vi "Andor_Measurement.vi"(5 "error in":errorcluster) -> (19 "error out":errorcluster)   [LabVIEW 2011]
uses:
  Program Files/National Instruments/LabVIEW 2011/resource/objmgr/daqmx.rc
  <vilib>/Utility/error.llb/DialogType.ctl
  Camera/lib/atmcd32d.llb/Error Code Enum typedef.ctl
  <vilib>/DAQmx/write.llb/DAQmx Write (Digital Bool 1Line 1Point).vi
  <vilib>/DAQmx/create/channels.llb/DAQmx Create Channel (DO-Digital Output).vi
  <vilib>/DAQmx/read.llb/DAQmx Read (Digital Bool 1Line 1Point).vi
  Kinetics/vi/GlobalSettings.vi
  Utilities/controls/ctlSeqFNs_PI_SysNr.ctl
  <vilib>/DAQmx/configure/trigger.llb/DAQmx Start Trigger (Digital Edge).vi
  <vilib>/DAQmx/create/channels.llb/DAQmx Create Channel (CO-Pulse Generation-Frequency).vi
  <vilib>/DAQmx/configure/timing.llb/DAQmx Timing (Implicit).vi
  <vilib>/DAQmx/create/channels.llb/DAQmx Create Channel (DI-Digital Input).vi
panel:
  in  "out":T1
  in  "valsZaxisMeasurement":T2
  out "error out 2":errorcluster
  out "last":i32
  out "first":u32
  out "pic2 2":dbl[][](graph)
  out "pic2":dbl[][](graph)
  out "intens":i32[][](graph)
  in  "PictureInfo 2":T3
  in  "Intensity DataInit":i32[][](graph)
  in  "Intensitätsdiode":dbl[](array[numeric])
  in  "Binning":T4
  in  "PictureInfo":T3
  out "y num vorgae":i32
  out "z vorgabe":i32
  out "z num":i32
  out "y num":i32
  out "x num":i32
  out "Intensity Graph Out Andor Null 2":i32[][](graph)
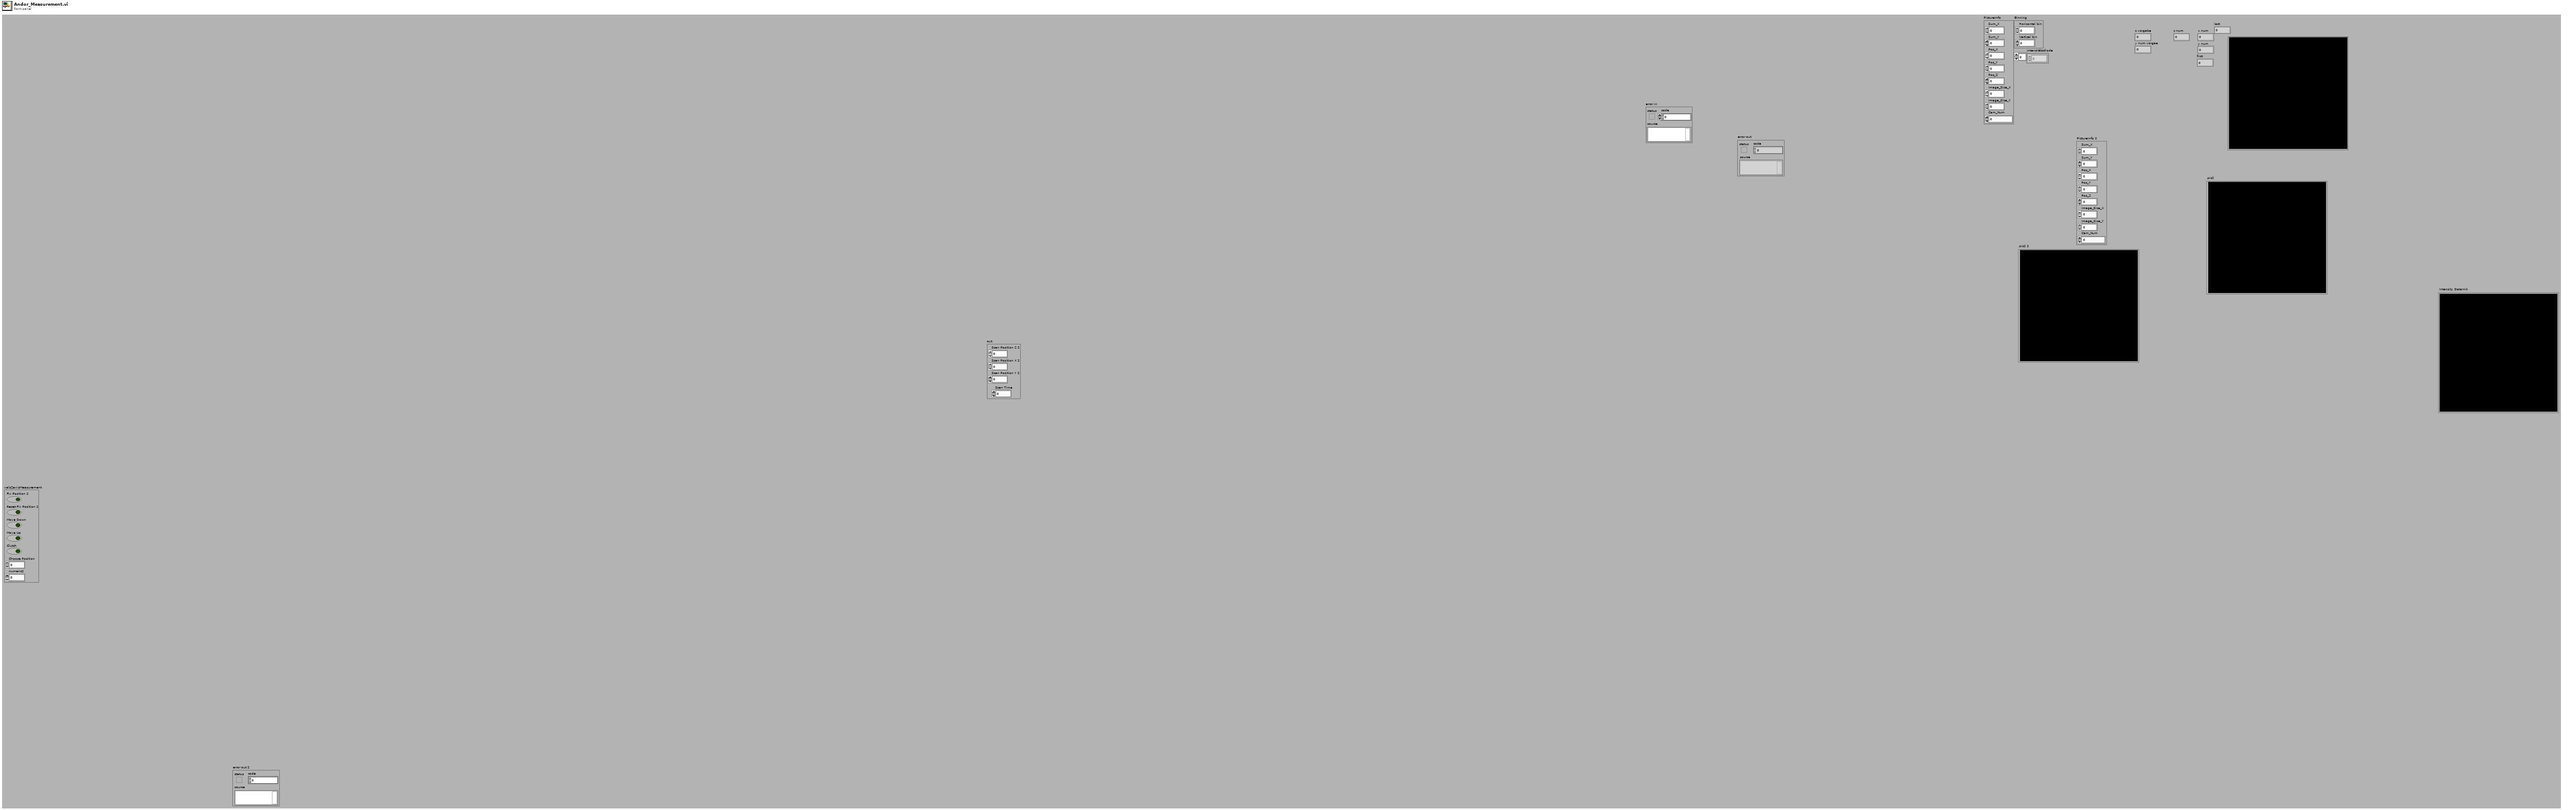
[diagram p1: front panel]
types:
  T1 = cluster{"Scan Position Z 2":dbl, "Scan Position X 2":dbl, "Scan Position Y 2":dbl, "Scan Time":dbl}
  T2 = cluster{"Fix Position 2":bool, "Reset Fix Position 2":bool, "Move Down":bool, "Move Up":bool, "Clutch":bool, "Choose Position":dbl, "numeric2":dbl}
  T3 = cluster{"Sum_X":i32, "Sum_Y":i32, "Pos_X":dbl, "Pos_Y":dbl, "Pos_Z":dbl, "Image_Size_X":dbl, "Image_Size_Y":dbl, "Cam_Num":i32}
  T4 = cluster{"Horizontal bin":i32, "Vertical bin":i32}
  T5 = typedef "ctlSeqFNs_PI_SysNr.ctl" = enum16{"Zero", "E517", "E710"}
  T6 = typedef "E517_Termination_character.ctl" = enum16{"LF", "CR", "LFCR", "CRLF"}
  T7 = typedef "E517_Controller_names.ctl" = enum16{"None", "Analog", "C-702", "C-843", "C-843.PM", "C-844", "C-848", "C-865", "C-866", "C-867", "C-880", "E-516", "E-517", "E-710", "E-712", "E-725", "E-753", "E-755", "E-761", "E-816", "E-861", "F-206", "M-840", "M-850", "M-8X0", "Mercury"}
  T8 = typedef "E517_Available_DLLs.ctl" = u16
  T9 = typedef "E517_Available_DLL_interfaces.ctl" = u16
  T10 = typedef "E517_Available_interfaces.ctl" = u16
  T11 = cluster{"Main-Global-Config out":cluster{"Global-Config":cluster{"DLL device ID's":i32[], "DLL Interface\nConfiguration":cluster{"DLL for Device":T8, "DLL Interface":T9, "Parameter":string}[], "Interface configuration":cluster{"RS232 Portnumber":i32, "Timeout":i32, "RS232 Baud rate":u32, "Interface":T10, "GPIB Bus":i32, "GPIB Address":i32, "GPIB Mode":i32}[], "Flow control":cluster{"input XON/XOFF":bool, "input HW Handshake":bool, "input alt HW HShk":bool, "output XON/XOFF":bool, "output HW Handshake":bool, "output alt HW HShk":bool, "XOFF byte ":u8, "XON byte":u8, "parity error byte":u16}[], "Bit settings and parity":cluster{"data bits":u16, "stop bits":enum16{"1 bit", "1.5 bits", "2 bits"}, "parity":enum16{"no parity", "odd parity", "even parity", "mark parity", "space parity"}}[], "TCP/IP Configuration":cluster{"Host address/name":string, "Port":i32, "Board":i32}[], "VISA Resource name":refnum<visa-resource-name>[], "Termination character":T6[], "Syntax":enum16{"GCS 1.0", "GCS 2.0"}[], "Logging mode":bool[], "Log file ref. no":refnum<file>[], "System no.":i32}, "DaisyChain configuration":cluster{"No. of devices":i32, "Port ID":i32, "Devices":string[], "Description":string}[], "System":cluster{"Conn. axes":string[], "Controller name":T7}[]}, "Axis-Status":cluster{"Online status (Array)?":bool[], "WG running?":bool[], "Servo status?":bool[]}, "Identification":string, "Conn. Axes":string[], "Position":dbl[], "+/- movement range":dbl[]}
  T12 = typedef "Error Code Enum typedef.ctl" = enum32{"N/A (0)", "DRV_ERROR_CODES", "DRV_SUCCESS", "DRV_VXDNOTINSTALLED", "DRV_ERROR_SCAN", "DRV_ERROR_CHECK_SUM", "DRV_ERROR_FILELOAD", "DRV_UNKNOWN_FUNC", "DRV_ERROR_VXD_INIT", "DRV_ERROR_ADDRESS", "DRV_ERROR_PAGELOCK", "DRV_ERROR_PAGEUNLOCK", "DRV_ERROR_BOARDTEST", "DRV_ERROR_ACK", "DRV_ERROR_UP_FIFO", "DRV_ERROR_PATTERN", "N/A (16)", "DRV_ACQUISITION_ERRORS", "DRV_ACQ_BUFFER", "DRV_ACQ_DOWNFIFO_FULL", "DRV_PROC_UNKONWN_INSTRUCTION", "DRV_ILLEGAL_OP_CODE", "DRV_KINETIC_TIME_NOT_MET", "DRV_ACCUM_TIME_NOT_MET", "DRV_NO_NEW_DATA", "N/A (25)", "DRV_SPOOLERROR", "N/A (27)", "N/A (28)", "N/A (29)", "N/A (30)", "N/A (31)", "N/A (32)", "DRV_TEMPERATURE_CODES", "DRV_TEMPERATURE_OFF", "DRV_TEMPERATURE_NOT_STABILIZED", "DRV_TEMPERATURE_STABILIZED", "DRV_TEMPERATURE_NOT_REACHED", "DRV_TEMPERATURE_OUT_RANGE", "DRV_TEMPERATURE_NOT_SUPPORTED", "DRV_TEMPERATURE_DRIFT", "N/A (41)", "N/A (42)", "N/A (43)", "N/A (44)", "N/A (45)", "N/A (46)", "N/A (47)", "N/A (48)", "DRV_GENERAL_ERRORS", "DRV_INVALID_AUX", "DRV_COF_NOTLOADED", "DRV_FPGAPROG", "DRV_FLEXERROR", "DRV_GPIBERROR", "N/A (55)", "N/A (56)", "N/A (57)", "N/A (58)", "N/A (59)", "N/A (60)", "N/A (61)", "N/A (62)", "N/A (63)", "DRV_DATATYPE", "DRV_DRIVER_ERRORS", "DRV_P1INVALID", "DRV_P2INVALID", "DRV_P3INVALID", "DRV_P4INVALID", "DRV_INIERROR", "DRV_COFERROR", "DRV_ACQUIRING", "DRV_IDLE", "DRV_TEMPCYCLE", "DRV_NOT_INITIALIZED", "DRV_P5INVALID", "DRV_P6INVALID", "DRV_INVALID_MODE", "DRV_INVALID_FILTER", "DRV_I2CERRORS", "DRV_I2CDEVNOTFOUND", "DRV_I2CTIMEOUT", "DRV_P7INVALID", "N/A (84)", "N/A (85)", "N/A (86)", "N/A (87)", "N/A (88)", "N/A (89)", "DRV_IOCERROR", "DRV_VRMVERSIONERROR"}
  T13 = cluster{"exposure":sgl, "accumulate":sgl, "kinetic":sgl}[]
  T14 = cluster{"exposure":sgl, "accumulate":sgl, "kinetic":sgl}
  T15 = cluster{"Initial delay":dbl, "Duty Cycle":dbl, "Frequency":dbl, "sample mode":i32, "Number Of Pulses":i32, "SrcToCtrOutTriggerForCamera":tag, "CtrOutTriggerForCamera":tag}
  T16 = cluster{"X-Min":dbl, "X-Len":dbl, "Y-Min":dbl, "Y-Len":dbl, "X-Delta":dbl, "Y-Delta ":dbl}
  T17 = cluster{"3d Layers_Num":dbl, "3d Start_Pos  Start":dbl, "3d Step_Delta_Layer":dbl}
  T18 = cluster{"Picture_Parameter_Out":enum16{"Maximized", "Averaged", "Normalized"}, "SavingMode":enum32{"Confocal", "HighRes", "Video", "Picture", "IntensityTrace", "Test"}}
  T19 = enum32{"Confocal", "HighRes", "Video", "Picture", "IntensityTrace", "Test"}
  T20 = typedef "DialogType.ctl" = u16
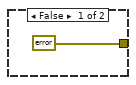
[diagram p3: hidden frame]
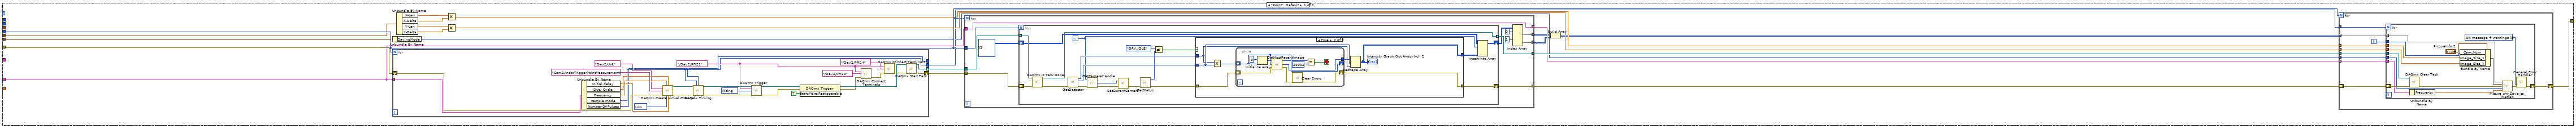
[diagram p4: hidden frame]
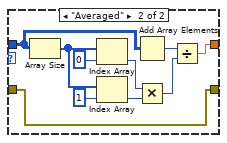
[diagram p9: hidden frame]
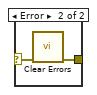
[diagram p10: hidden frame]
diagram:
  (unwired) ctlSeqFNs_PI_SysNr."E710" ("DeviceNr.")
  n1 = case shown="\"Point\", Default" {
    selector: _ -> [_ _]
    tunnel: _ -> [w45 _]
    tunnel: [w39 w46] -> w12
    tunnel: _ -> [w44 _]
    tunnel: [w42 _] -> w4
    frame "Point", Default {
      n2 = Unbundle By Name(w44) -> ("Conn. Axes"=w43)
      n3 = call "MVR.vi"("System no."=w42, "Axes to move"=w43, "Position values"=dbl[] [100.0, 100.0], "No.of digits"=i16 4, "error in"=w45) -> ("error out"=w39:errorcluster)  [unwired: 14 in]
    }
    frame "XDArea" {
    }
  }
  "error out 2" <- w12
  n4 = call "MeasurementAktivFCG.vi"("error in"="error in", "Set_Get"=enum16{"Set", "Get"}."Set", "Value"=TRUE) -> ("error out"=w9:errorcluster)  [unwired: 7 in, 1 out]
  n5 = call "HeidenhainValsPre.vi"(1:"valsZaxisMeasurement", 2:TRUE ("Reset Fix Position"), 5:w9) -> (6:w3)  [unwired: 5 in]
  n6 = call "SetupAquisitionParameters.vi"("error in"=w3) -> ("error out"=w13:errorcluster)  [unwired: 18 in]
  n7 = call "SetGetMeasurement_TypeFGV.vi"("error in"=w13, "FGV_Control"=enum16{"Set", "Get"}."Get") -> ("error out"=w20:errorcluster, "Measurement Type 2"=w22:enum16{"Point", "XDArea"})  [unwired: 8 in]
  n8 = call "ConfigureCamera.vi"("error in"=w20, "Set_Get"=enum16{"Set", "Get"}."Get") -> ("error out"=w19:errorcluster, "out"=w17:cluster{"Hbin":i32, "Vbin":i32, "ExpTime":sgl})  [unwired: 8 in]
  n9 = Unbundle By Name(w17) -> ("Vbin"=w16:i32, "Hbin"=w15:i32)
  n10 = call "GetAvailableCameras.vi"("error in (no error)"=w19) -> ("error out"=w25:errorcluster, "totalCameras"=w14:i32, "DLL error code"=w37:u32)  [unwired: 2 in]
  n11 = call "SetAndorOnlineOfflineFGV.vi"("error in"=w25, "Set_Get"=enum16{"Set", "Get"}."Get") -> ("error out"=w6:errorcluster, "andor 1"=w29:bool, "andor 0"=w30:bool)  [unwired: 7 in]
  n12 = Not(x=w30) -> (.not. x?=w27:bool)
  n13 = global read "GlobalSettings.vi" "scanner global out"() -> (w5:T11)
  n14 = Boolean To (0,1)(Boolean=w27) -> (0, 1=w31:i16)
  n15 = Not(x=w29) -> (.not. x?=w28:bool)
  n16 = Subtract(x=w14, y=w31) -> (x-y=w32:i32)
  n17 = Boolean To (0,1)(Boolean=w28) -> (0, 1=w33:i16)
  n18 = Subtract(x=w32, y=w33) -> (x-y=w23:i32)
  n19 = Not Equal To 0?(x=w23) -> (x != 0?=w34:bool)
  n20 = Equal?(x=w37, y=u32 20002) -> (x = y?=w35:bool)
  n21 = Or(x=w34, y=w35) -> (x .or. y?=w24:bool)
  n22 = case shown="True" w24 {
    tunnel: w23 -> [_ w79]
    tunnel: w22 -> [_ w72]
    tunnel: [errorcluster {"status"=FALSE, "code"=0, "source"="noCameraAtSetupAcquisitionParameters"} ("error out") w78] -> w21
    tunnel: w16 -> [_ w65]
    tunnel: w15 -> [_ w64]
    tunnel: w6 -> [_ w51]
    tunnel: w5 -> [_ w48]
    tunnel: ctlSeqFNs_PI_SysNr."E710" ("DeviceNr.") -> [_ w49]
    frame False {
    }
    frame True {
      n23 = call "GetConfiguratioOfCamera.vi"("error in"=w51, "Set_Get"=enum16{"Set", "Get"}."Get") -> ("error out"=w62:errorcluster, "out"=w55:T13)  [unwired: 8 in]
      n24 = Index Array(array=w55, index #1=0 ("index"), index #2=1 ("index")) -> (element #1=w58:T14, element #2=w59:T14)
      n25 = Unbundle By Name(w58) -> ("exposure"=w60:sgl)
      n26 = Unbundle By Name(w59) -> ("exposure"=w61:sgl)
      n27 = Max & Min(x=w60, y=w61) -> (max(x,y)=w50:sgl)  [unwired: 1 out]
      n28 = call "3D_Distance_FGV.vi"("error in"=w62, "FGV_Control"=enum16{"Set", "Get"}."Get") -> ("error out"=w52:errorcluster)  [unwired: 8 in, 1 out]
      n29 = call "TriggerPointMeasurement.vi"("error in"=w52, "Set_Get"=enum16{"Set", "Get"}."Get") -> ("error out"=w75:errorcluster, "out"=w76:T15)  [unwired: 8 in]
      n30 = call "RoiSelectionCoordinates.vi"("error in"=w75, "FGV_Control"=enum16{"Set", "Get"}."Get") -> ("error out"=w71:errorcluster, "ROI Coordinates out"=w73:T16)  [unwired: 8 in]
      n31 = call "3D_Distance_FGV.vi"("error in"=w71, "FGV_Control"=enum16{"Set", "Get"}."Get") -> ("error out"=w68:errorcluster, "3D out"=w69:T17)  [unwired: 8 in]
      n32 = call "Save_Picture_Parameter_FGV.vi"("error in"=w68, "FGV_Control"=enum16{"Set", "Get"}."Get") -> ("error out"=w63:errorcluster, "Picture_Parameter_Out"=w66:T18)  [unwired: 8 in]
      n33 = case shown="\"XDArea\"" w72 {
        tunnel: w79 -> [w95 w324]
        tunnel: [w101 w261] -> w78
        tunnel: w63 -> [w99 w209]
        tunnel: w76 -> [w94 _]
        tunnel: w73 -> [w90 w210]
        tunnel: w69 -> [_ w207]
        tunnel: w66 -> [w92 w302]
        tunnel: w65 -> [_ w292]
        tunnel: w64 -> [_ w293]
        tunnel: w50 -> [_ w208]
        tunnel: w49 -> [_ w206]
        tunnel: w48 -> [_ w205]
        frame "Point", Default {
          n34 = Unbundle By Name(w92) -> ("SavingMode"=w91:T19)
          n35 = for {
            N: w95 -> [_]
            shift-right: [w188] -> w100
            shift-left: w99 -> [w176]
            tunnel: w94 -> [w186]
            tunnel: [w187] -> w98 mode=indexing
            tunnel: [w178] -> w80
            tunnel: [w177] -> _
            w180 = tag "/Dev2/PFI21" ("source")
            w197 = 10280 items=["Rising"=10280, "Falling"=10171] ("Trigger Edge")
            w200 = 10214 items=["High"=10192, "Low"=10214] ("Idle State")
            n36 = Unbundle By Name(w186) -> ("Initial delay"=w189:dbl, "Duty Cycle"=w191:dbl, "Frequency"=w190:dbl, "sample mode"=w177:i32, "Number Of Pulses"=w178:i32)
            n37 = call-poly <vilib>:"DAQmx Create Virtual Channel.vi"("frequency"=w190, "duty cycle"=w191, "counter"=tag "Dev2/ctr6", "name to assign"="Cam1AndorTriggerPointMeasurement", "error in"=w176, "idle state"=w200, "initial delay"=w189) -> ("task out"=w201:refnum<k21>, "error out"=w202:errorcluster)  [unwired: 7 in]
            n38 = call-poly <vilib>:"DAQmx Timing.vi"("task/channels in"=w201, "sample mode"=w177, "samples per channel"=w178, "error in"=w202) -> ("task out"=w199:refnum<k21>, "error out"=w198:errorcluster)  [unwired: 10 in]
            n39 = call-poly <vilib>:"DAQmx Trigger.vi"("task/channels in"=w199, "source"=w180, "edge"=w197, "error in"=w198) -> ("task out"=w195:refnum<k21>, "error out"=w194:errorcluster)  [unwired: 10 in]
            n40 = property class="DAQmx Trigger"(reference=w195, error in=w194, "Start:More:Retriggerable"=TRUE) -> (reference out=w192:refnum<k21>, error out=w183:errorcluster)
            n41 = call <vilib>:"DAQmx Connect Terminals.vi"("source terminal"=w180, "destination terminal"=tag "/Dev2/PFI20", "error in"=w183) -> ("error out"=w182:errorcluster)  [unwired: 12 in]
            n42 = call <vilib>:"DAQmx Connect Terminals.vi"("source terminal"=w180, "destination terminal"=tag "/Dev2/PFI24", "error in"=w182) -> ("error out"=w181:errorcluster)  [unwired: 12 in]
            n43 = call <vilib>:"DAQmx Start Task.vi"("task/channels in"=w192, "error in"=w181) -> ("task out"=w187:refnum<k21>, "error out"=w188:errorcluster)  [unwired: 12 in]
          }
          n44 = Unbundle By Name(w90) -> ("X-Len"=w89:dbl, "X-Delta"=w88:dbl, "Y-Len"=w86:dbl, "Y-Delta"=w87:dbl)
          n45 = Multiply(x=w89, y=w88) -> (x*y=w85:dbl)
          n46 = Multiply(x=w86, y=w87) -> (x*y=w84:dbl)
          n47 = for {
            N: w80 -> [_]
            tunnel: w100 -> [w113]
            tunnel: w98 -> [w112]
            tunnel: [w111] -> w97
            tunnel: [w110] -> w96
            tunnel: w95 -> [w109]
            tunnel: w94 -> [w108]
            tunnel: [w108] -> w93
            tunnel: [w104] -> w83 mode=indexing
            tunnel: [w102] -> w82 mode=indexing
            n48 = for {
              N: w109 -> [_]
              shift-right: [w122] -> w111
              shift-left: w113 -> [w118]
              tunnel: [w119] -> w110 mode=indexing
              tunnel: w112 -> [w120] mode=indexing
              shift-right: [w116] -> w106
              shift-left: i32[][][] [] ("array") -> [w115]
              i -> [w117]
              n49 = call <vilib>:"DAQmx Is Task Done.vi"("task/channels in"=w120, "error in"=w118) -> ("task out"=w119:refnum<k21>, "error out"=w123:errorcluster)  [unwired: 11 in, 1 out]
              n50 = call "GetDetector.vi"("error in (no error)"=w123) -> ("error out"=w126:errorcluster, "ypixels"=w124:i32, "xpixels"=w125:i32)  [unwired: 3 in, 1 out]
              n51 = call "GetCameraHandle.vi"("error in (no error)"=w126, "cameraIndex"=w117) -> ("error out"=w131:errorcluster, "cameraHandle"=w132:i32)  [unwired: 1 in, 1 out]
              n52 = call "SetCurrentCamera.vi"("error in (no error)"=w131, "cameraHandle"=w132) -> ("error out"=w130:errorcluster)  [unwired: 1 out]
              n53 = call "GetStatus.vi"("error in (no error)"=w130) -> ("error out"=w129:errorcluster, "status"=w127:T12)  [unwired: 2 in, 1 out]
              n54 = Not Equal?(x=Error_Code_Enum_typedef."DRV_IDLE" ("status"), y=w127) -> (x != y?=w121:bool)
              n55 = case shown="True" w121 {
                tunnel: [w133 w134] -> w122
                tunnel: w129 -> [w133 w138]
                tunnel: w125 -> [_ w136]
                tunnel: w124 -> [_ w137]
                tunnel: [_ w135] -> w114
                frame False {
                }
                frame True {
                  n56 = Multiply(x=w136, y=w137) -> (x*y=w139:i32)
                  n57 = while {
                    tunnel: [w144] -> w140
                    shift-right: [w147] -> w134
                    shift-left: w138 -> [w141]
                    shift-right: [w145] -> _
                    shift-left: w139 -> [w145]
                    stop <- w149 stop-if-true
                    n58 = Initialize Array(0 ("element"), w145) -> (w146:i32[])
                    n59 = call "GetMostRecentImage.vi"("error in (no error)"=w141, "size"=w145, "array"=w146) -> ("error out"=w142:errorcluster, "array"=w144:i32[], "DLL error code"=w143:u32)
                    n60 = call <vilib>:"Clear Errors.vi"("error in (no error)"=w142) -> ("error out"=w147:errorcluster)  [unwired: 6 in]
                    n61 = Equal?(x=w143, y=u32 20002) -> (x = y?=w149:bool)
                  }
                  n62 = Reshape Array(w140, w137, w136) -> (w135:i32[][])
                  "Intensity Graph Out Andor Null 2" <- w135
                }
              }
              n63 = Insert Into Array(array=w115, index (dim 0)=w117, new element=w114) -> (w116:i32[][][])  [unwired: 2 in]
            }
            n64 = Index Array(array=w106, index (dim 0) #1=0 ("index"), index (dim 0) #2=1 ("index (page)")) -> (element #1=w104:i32[][], element #2=w102:i32[][])  [unwired: 4 in]
          }
          n65 = Build Array(w83, w82) -> (w81:i32[][][][])
          n66 = for {
            N: w95 -> [_]
            shift-right: [w151] -> w101
            shift-left: w97 -> [w160]
            tunnel: w96 -> [w159] mode=indexing
            tunnel: w93 -> [w158]
            tunnel: w91 -> [w157]
            tunnel: w85 -> [w155]
            tunnel: w84 -> [w154]
            tunnel: w81 -> [w153] mode=indexing
            tunnel: w80 -> [w152]
            i -> [w156]
            n67 = for {
              N: w152 -> [_]
              tunnel: w159 -> [w173]
              tunnel: w158 -> [w172]
              tunnel: w157 -> [w168]
              tunnel: w156 -> [w165]
              tunnel: w155 -> [w164]
              tunnel: w154 -> [w163]
              tunnel: w153 -> [w162] mode=indexing
              shift-right: [w161] -> w151
              shift-left: w160 -> [w174]
              w175 = T20 3 items=["no dialog", "OK message", "continue or stop message", "OK message + warnings", "continue/stop + warnings"] ("type of dialog (OK msg:1)")
              n68 = call <vilib>:"DAQmx Clear Task.vi"("task in"=w173, "error in"=w174) -> ("error out"=w171:errorcluster)  [unwired: 13 in]
              n69 = Unbundle By Name(w172) -> ("Frequency"=w169:dbl)
              n70 = Bundle By Name(cluster="PictureInfo 2", "Cam_Num"=w165, "Image_Size_X"=w164, "Image_Size_Y"=w163) -> (w166:T3)
              n71 = call "Picture_shr_Save_to_matlab.vi"("DataIn"=w162, "PictureInfo"=w166, "error in"=w171, "SavingMode"=w168, "Freuquency"=w169) -> ("error out"=w170:errorcluster)  [unwired: 10 in]
              n72 = call <vilib>:"General Error Handler.vi"("type of dialog (OK msg:1)"=w175, "error in (no error)"=w170) -> ("error out"=w161:errorcluster)  [unwired: 9 in, 4 out]
            }
          }
        }
        frame "XDArea" {
          w217 = 0 ("X0")
          w252 = TRUE ("All axes?")
          w307 = T20 0 items=["no dialog", "OK message", "continue or stop message", "OK message + warnings", "continue/stop + warnings"] ("type of dialog (OK msg:1)")
          w312 = T20 0 items=["no dialog", "OK message", "continue or stop message", "OK message + warnings", "continue/stop + warnings"] ("type of dialog (OK msg:1)")
          n73 = Unbundle By Name(w210) -> ("X-Min"=w222:dbl, "Y-Min"=w245:dbl, "X-Len"=w218:dbl, "Y-Len"=w250:dbl, "Y-Delta"=w248:dbl, "X-Delta"=w223:dbl)
          n74 = Divide(x=w250, y=w248) -> (x/y=w249:dbl)
          n75 = Divide(x=w218, y=w223) -> (x/y=w221:dbl)
          n76 = call "Calc_frequency.vi"("ExitationTime In"=w208, "X-length"=w218, "CamTolerance"=1.1, "frequency in"=5000, "error in"=w209, "X-Delta"=w223) -> ("Wavepoints"=w212:dbl, "N"=w211:dbl, "TriggerLineCamWavepoints"=w216:dbl[], "divisor out"=w215:i32, "Array"=w214:u8[], "error out"=w220:errorcluster)  [unwired: 4 in]
          n77 = Unbundle By Name(w205) -> ("Conn. Axes"=w213:string[])
          n78 = call "Calc_WaveformGenerator.vi"("Scan parameters"=w215, "Wavepoint"=w213, "Trigger value 2"=w212, 3:w214, "wave table rate/ms"=w217, "System no."=w206, "scan time for 1 line/ms"=w217, 7:w216, 8:w211, 9:w217, 10:w211, "error in 2"=w220, 12:w218) -> ("error out 2"=w219:errorcluster)  [unwired: 2 in]
          n79 = call "ONT?.vi"("System no."=w206, "Axes to query"=w213, "All axes?"=w252, "Axis identifier?"=w252, "error in"=w219) -> ("error out"=w257:errorcluster)  [unwired: 13 in, 1 out]
          n80 = call "TMN?.vi"("System no."=w206, "Axes to query"=w213, "All axes?"=w252, "Axis identifier?"=w252, "error in"=w257) -> ("error out"=w258:errorcluster)  [unwired: 13 in, 1 out]
          n81 = call "TMX?.vi"("System no."=w206, "Axes to query"=w213, "All axes?"=w252, "Axis identifier?"=w252, "error in"=w258) -> ("error out"=w253:errorcluster)  [unwired: 13 in, 1 out]
          n82 = for {
            N: w249 -> [_]
            shift-right: [w398] -> _
            shift-left: w245 -> [w399]
            tunnel: [w398] -> w256 mode=indexing
            shift-right: [w397] -> w254
            shift-left: w253 -> [w397]
            tunnel: w248 -> [w396]
            n83 = Add(x=w399, y=w396) -> (x+y=w398:dbl)
          }
          n84 = Unbundle By Name(w207) -> ("3d Layers_Num"=w251:dbl, "3d Start_Pos  Start"=w244:dbl, "3d Step_Delta_Layer"=w247:dbl)
          n85 = Divide(x=w251, y=w247) -> (x/y=w246:dbl)
          n86 = for {
            N: w246 -> [_]
            shift-right: [w394] -> _
            shift-left: w244 -> [w395]
            tunnel: [w394] -> w255 mode=indexing
            shift-right: [w393] -> w243
            shift-left: w254 -> [w393]
            tunnel: w247 -> [w392]
            n87 = Add(x=w395, y=w392) -> (x+y=w394:dbl)
          }
          n88 = Unbundle By Name(w302) -> ("Picture_Parameter_Out"=w269:enum16{"Maximized", "Averaged", "Normalized"}, "SavingMode"=w296:T19)
          n89 = Unbundle By Name(w207) -> ("3d Step_Delta_Layer"=w277:dbl, "3d Layers_Num"=w279:dbl, "3d Start_Pos  Start"=w270:dbl)
          n90 = call "StartTimingDIO_ScannerStage.vi"(2:w243) -> (5:w240, 7:w239, 11:w241, 13:w234, 14:w237, 15:w235, 16:w204, 17:w236, 18:w242, 19:w238)  [unwired: 9 in]
          n91 = Divide(x=w279, y=w277) -> (x/y=w278:dbl)
          n92 = for {
            N: w246 -> [_]
            tunnel: w213 -> [w350]
            tunnel: w206 -> [w349]
            tunnel: w256 -> [w348]
            tunnel: w222 -> [w347]
            tunnel: w255 -> [w346] mode=indexing
            shift-right: [w345] -> w233
            shift-left: _ -> [_]
            tunnel: w249 -> [w344]
            tunnel: w242 -> [w343]
            tunnel: w241 -> [w342]
            tunnel: w240 -> [w341]
            tunnel: w239 -> [w340]
            tunnel: w238 -> [w339]
            tunnel: w237 -> [w338]
            tunnel: w236 -> [w337]
            tunnel: w235 -> [w336]
            tunnel: w234 -> [w335]
            tunnel: [w334] -> w232
            tunnel: [w333] -> w231
            tunnel: [w332] -> w230
            tunnel: [w331] -> w229
            tunnel: [w330] -> w228
            tunnel: [w329] -> w227
            tunnel: [w328] -> w226
            tunnel: [w327] -> w225
            tunnel: [w326] -> w224
            tunnel: w221 -> [w325]
            n93 = for {
              N: w344 -> [_]
              shift-right: [_] -> w345
              shift-left: _ -> [_]
              tunnel: w349 -> [w352]
              tunnel: w350 -> [w353]
              tunnel: w348 -> [w389] mode=indexing
              tunnel: w347 -> [w388]
              tunnel: w346 -> [w387]
              tunnel: w343 -> [w372]
              tunnel: w342 -> [w371]
              tunnel: w341 -> [w370]
              tunnel: w340 -> [w369]
              tunnel: w339 -> [w368]
              tunnel: w338 -> [w367]
              tunnel: w337 -> [w366]
              tunnel: w336 -> [w365]
              tunnel: w335 -> [w364]
              tunnel: [w363] -> w334
              tunnel: [w362] -> w333
              tunnel: [w361] -> w332
              tunnel: [w360] -> w331
              tunnel: [w359] -> w330
              tunnel: [w358] -> w329
              tunnel: [w357] -> w328
              tunnel: [w356] -> w327
              tunnel: [w355] -> w326
              tunnel: w325 -> [w354]
              w385 = TRUE ("Axis identifier?")
              n94 = Build Array(w388, w389, w387) -> (w390:dbl[])
              n95 = call "MOV.vi"("System no."=w352, "Axes to move"=w353, "Position values"=w390, "No.of digits"=i16 1) -> ("error out"=w351:errorcluster)  [unwired: 15 in]
              n96 = call "TriggerTheCamera.vi"(0:w372, 1:w368, 2:w367, 3:w366, 4:w365, 5:w364, 6:w354, "error out 2"=w351, 8:w371, 10:w370, 12:w369) -> (14:w355, 16:w356, 18:w357, 21:w358, 22:w359, 23:w360, 24:w361, 25:w362, 26:w363, "error out"=w386:errorcluster)  [unwired: 7 in]
              n97 = call "POS?.vi"("System no."=w352, "Axes to query"=w353, "All axes?"=w385, "Axis identifier?"=w385, "error in"=w386) -> ("Position"=w380:dbl[], "error out"=w384:errorcluster)  [unwired: 13 in]
              n98 = Index Array(array=w380, index #1=0 ("index"), index #2=1 ("index"), index #3=2 ("index")) -> (element #1=w378:dbl, element #2=w376:dbl, element #3=w374:dbl)
              n99 = Bundle By Name(cluster="out", "Scan Position X 2"=w378, "Scan Position Y 2"=w376, "Scan Position Z 2"=w374) -> (w381:T1)
              n100 = call "ScanPosition_FGV.vi"("error in"=w384, "FGV_Control"=enum16{"Set", "Get"}."Set", "in"=w381) -> ("error out"=w383:errorcluster)  [unwired: 7 in, 1 out]
              n101 = call <vilib>:"Clear Errors.vi"("error in (no error)"=w383) -> ()  [unwired: 6 in, 1 out]
            }
          }
          n102 = call-poly <vilib>:"DAQmx Create Virtual Channel.vi"("lines"=tag "Dev2/port0/line10", "name to assign"="CamStartInputTimer", "error in"=w204) -> ("task out"=w287:refnum<k21>, "error out"=w265:errorcluster)  [unwired: 11 in]
          n103 = call-poly <vilib>:"DAQmx Create Virtual Channel.vi"("lines"=tag "Dev2/port0/line5", "name to assign"="CameraStartInput", "error in"=w265) -> ("task out"=w316:refnum<k21>, "error out"=w321:errorcluster)  [unwired: 11 in]
          n104 = call-poly <vilib>:"DAQmx Create Virtual Channel.vi"("lines"=tag "Dev2/port0/line6", "name to assign"="CameraReadOutDoneX", "error in"=w321) -> ("task out"=w314:refnum<k21>, "error out"=w306:errorcluster)  [unwired: 11 in]
          n105 = call <vilib>:"DAQmx Start Task.vi"("task/channels in"=w316, "error in"=w306) -> ("task out"=w315:refnum<k21>, "error out"=w266:errorcluster)  [unwired: 12 in]
          n106 = call <vilib>:"DAQmx Start Task.vi"("task/channels in"=w287, "error in"=w266) -> ("task out"=w286:refnum<k21>, "error out"=w267:errorcluster)  [unwired: 12 in]
          n107 = call-poly <vilib>:"DAQmx Write.vi"("task/channels in"=w286, "data"=FALSE, "error in"=w267) -> ("task out"=w285:refnum<k21>, "error out"=w280:errorcluster)  [unwired: 10 in, 1 out]
          n108 = Unbundle By Name(w210) -> ("X-Min"=w275:dbl, "Y-Min"=w298:dbl, "X-Len"=w273:dbl, "Y-Len"=w271:dbl, "X-Delta"=w276:dbl, "Y-Delta"=w281:dbl)
          n109 = call "CameraReady.vi"("error in"=w280, "Set_Get"=enum16{"Set", "Get"}."Set", "Value"=TRUE) -> ("error out"=w203:errorcluster)  [unwired: 7 in, 1 out]
          n110 = Divide(x=w273, y=w276) -> (x/y=w274:dbl)
          n111 = Divide(x=w271, y=w281) -> (x/y=w272:dbl)
          n112 = for {
            N: w278 -> [w441]
            tunnel: w324 -> [w443]
            tunnel: w272 -> [w434]
            tunnel: w274 -> [w442]
            shift-right: [w431] -> w310
            shift-left: w203 -> [w436]
            tunnel: w315 -> [w440]
            tunnel: w314 -> [w439]
            tunnel: [w438] -> w308
            tunnel: [w437] -> w309
            tunnel: [w435] -> w300
            tunnel: [w434] -> w299
            tunnel: [w433] -> w305
            tunnel: w269 -> [w432]
            tunnel: w285 -> [w425]
            tunnel: [w426] -> w284
            tunnel: [w421] -> w264 mode=indexing
            tunnel: [w420] -> w263 mode=indexing
            i -> [w433]
            n113 = for {
              N: w434 -> [w498]
              tunnel: w443 -> [w506]
              shift-right: [w504] -> w429
              shift-left: w436 -> [w483]
              tunnel: w440 -> [w505]
              tunnel: w439 -> [w496]
              tunnel: [w493] -> w438
              tunnel: [w503] -> w437
              tunnel: w442 -> [w502]
              tunnel: [w492] -> w435
              tunnel: w432 -> [w491]
              tunnel: [w490] -> w430
              tunnel: w425 -> [w481]
              tunnel: [w489] -> w426
              tunnel: [w488] -> w424
              tunnel: [w487] -> w423
              tunnel: [w469] -> w421 mode=indexing
              tunnel: [w468] -> w420 mode=indexing
              i -> [w473]
              n114 = call-poly <vilib>:"DAQmx Write.vi"("task/channels in"=w481, "data"=FALSE, "error in"=w483) -> ("task out"=w482:refnum<k21>, "error out"=w478:errorcluster)  [unwired: 10 in, 1 out]
              n115 = call-poly <vilib>:"DAQmx Write.vi"("task/channels in"=w496, "data"=FALSE, "timeout"=10.0, "error in"=w478) -> ("task out"=w495:refnum<k21>, "error out"=w497:errorcluster)  [unwired: 9 in, 1 out]
              n116 = while {
                tunnel: w497 -> [w511]
                tunnel: w505 -> [w515]
                tunnel: [w514] -> w499
                tunnel: w482 -> [w513]
                tunnel: [w512] -> w485
                tunnel: [w509] -> w477
                stop <- w507 stop-if-true
                n117 = call-poly <vilib>:"DAQmx Read.vi"("task/channels in"=w515, "error in"=w511) -> ("task out"=w514:refnum<k21>, "data"=w507:bool, "error out"=w510:errorcluster)  [unwired: 11 in]
                n118 = call-poly <vilib>:"DAQmx Write.vi"("task/channels in"=w513, "data"=TRUE, "error in"=w510) -> ("task out"=w512:refnum<k21>, "error out"=w509:errorcluster)  [unwired: 10 in, 1 out]
              }
              n119 = call-poly <vilib>:"DAQmx Write.vi"("task/channels in"=w485, "data"=FALSE, "error in"=w477) -> ("task out"=w486:refnum<k21>, "error out"=w484:errorcluster)  [unwired: 10 in, 1 out]
              n120 = for {
                N: w506 -> [_]
                shift-right: [w519] -> w500
                shift-left: w484 -> [w537]
                tunnel: w495 -> [w535]
                tunnel: [w536] -> w493
                tunnel: w499 -> [w536]
                tunnel: [w535] -> w494
                tunnel: w502 -> [w516]
                tunnel: [w516] -> w492
                tunnel: w491 -> [w534]
                tunnel: [w529] -> w490 mode=indexing
                tunnel: w486 -> [w533]
                tunnel: [w533] -> w489
                tunnel: [w532] -> w488
                tunnel: [w531] -> w487
                tunnel: [w530] -> w472 mode=indexing
                i -> [w529]
                n121 = call "GetDetector.vi"("error in (no error)"=w537) -> ("error out"=w540:errorcluster, "ypixels"=w538:i32, "xpixels"=w539:i32)  [unwired: 3 in, 1 out]
                n122 = Multiply(x=w539, y=w538) -> (x*y=w526:i32)
                n123 = call "GetCameraHandle.vi"("error in (no error)"=w540, "cameraIndex"=w529) -> ("error out"=w544:errorcluster, "cameraHandle"=w545:i32)  [unwired: 1 in, 1 out]
                n124 = call "SetCurrentCamera.vi"("error in (no error)"=w544, "cameraHandle"=w545) -> ("error out"=w543:errorcluster)  [unwired: 1 out]
                n125 = call "GetStatus.vi"("error in (no error)"=w543) -> ("error out"=w522:errorcluster, "status"=w541:T12)  [unwired: 2 in, 1 out]
                n126 = Not Equal?(x=Error_Code_Enum_typedef."DRV_IDLE" ("status"), y=w541) -> (x != y?=w523:bool)
                n127 = case shown="True" w523 {
                  tunnel: [w546 w547] -> w521
                  tunnel: w522 -> [w546 w548]
                  frame False {
                  }
                  frame True {
                    n128 = call "AbortAcquisition.vi"("error in (no error)"=w548) -> ("error out"=w547:errorcluster)  [unwired: 1 in, 1 out]
                  }
                }
                n129 = call "GetNumberNewImages.vi"("error in (no error)"=w521) -> ("error out"=w528:errorcluster, "last"=→"last":i32, "first"=→"first":u32)  [unwired: 3 in, 1 out]
                n130 = for {
                  N: w516 -> [_]
                  tunnel: w526 -> [w561]
                  tunnel: w528 -> [w560]
                  tunnel: [w556] -> w525
                  tunnel: w538 -> [w553]
                  tunnel: w539 -> [w552]
                  shift-right: [w551] -> _
                  shift-left: i32[][][] [] ("output array") -> [w558]
                  tunnel: [w555] -> w530 mode=indexing
                  tunnel: w534 -> [w554]
                  tunnel: [w553] -> w532
                  tunnel: [w552] -> w531
                  i -> [w549]
                  n131 = while {
                    tunnel: [w576] -> w559
                    shift-right: [w583] -> w557
                    shift-left: w560 -> [w579]
                    shift-right: [w582] -> _
                    shift-left: w561 -> [w582]
                    stop <- w577 stop-if-true
                    n132 = Initialize Array(0 ("element"), w582) -> (w575:i32[])
                    n133 = call "GetOldestImage.vi"("error in (no error)"=w579, "size"=w582, "array"=w575) -> ("error out"=w580:errorcluster, "array"=w576:i32[], "DLL error code"=w581:u32)
                    n134 = call <vilib>:"Clear Errors.vi"("error in (no error)"=w580) -> ("error out"=w583:errorcluster)  [unwired: 6 in]
                    n135 = Equal?(x=w581, y=u32 20002) -> (x = y?=w577:bool)
                  }
                  n136 = Reshape Array(w559, w553, w552) -> (w550:i32[][])
                  "intens" <- w550
                  n137 = Insert Into Array(array=w558, index (dim 0)=w549, new element=w550) -> (w551:i32[][][])  [unwired: 2 in]
                  n138 = case shown="\"Maximized\", Default" w554 {
                    tunnel: [w562 w573] -> w555
                    tunnel: w551 -> [w564 w566]
                    tunnel: w557 -> [w563 w565]
                    tunnel: [w563 w565] -> w556
                    frame "Maximized", Default {
                      n139 = Array Max & Min(array=w564) -> (max value=w562:i32)  [unwired: 3 out]
                    }
                    frame "Averaged" {
                      n140 = Array Size(array=w566) -> (size(s)=w570:i32[])
                      n141 = Index Array(array=w570, index=0 ("Index")) -> (element=w568:i32)
                      n142 = Index Array(array=w570, index=1 ("Index")) -> (element=w567:i32)
                      n143 = Add Array Elements(numeric array=w566) -> (sum=w574:i32)
                      n144 = Multiply(x=w568, y=w567) -> (x*y=w569:i32)
                      n145 = Divide(x=w574, y=w569) -> (x/y=w573:dbl)
                    }
                  }
                  "x num" <- w549
                }
                n146 = case shown="No Error" w525 {
                  selector: w525 -> [w585 w587]
                  tunnel: [w585 w586] -> w517
                  frame No Error {
                  }
                  frame Error {
                    n147 = call <vilib>:"Clear Errors.vi"("error in (no error)"=w587) -> ("error out"=w586:errorcluster)  [unwired: 6 in]
                  }
                }
                n148 = call "FreeInternalMemory.vi"("error in (no error)"=w517) -> ("error out"=w520:errorcluster)  [unwired: 1 in, 1 out]
                n149 = call "StartAcquisition.vi"("error in (no error)"=w520) -> ("error out"=w519:errorcluster)  [unwired: 1 in, 1 out]
              }
              n150 = call-poly <vilib>:"DAQmx Write.vi"("task/channels in"=w494, "auto start"=TRUE, "data"=TRUE, "error in"=w500) -> ("task out"=w503:refnum<k21>, "error out"=w504:errorcluster)  [unwired: 9 in, 1 out]
              n151 = Index Array(array=w472, index (row) #1=0 ("index (row)"), index (row) #2=1 ("index (row)")) -> (element #1=w469:dbl[], element #2=w468:dbl[])  [unwired: 2 in]
              "y num" <- w473
              "y num vorgae" <- w498
            }
            "pic2" <- w421
            "pic2 2" <- w420
            n152 = call "Measurement_Check_FGV.vi"("error in"=w429, "FGV_Control"=enum16{"Set", "Get"}."Get") -> ("error out"=w428:errorcluster, "Measurement_Preview_Out"=w422:bool)  [unwired: 8 in]
            n153 = case shown="True" w422 {
              tunnel: [w444 w451] -> w431
              tunnel: w428 -> [w444 w448]
              tunnel: w423 -> [_ w450]
              tunnel: w430 -> [_ w449]
              tunnel: w424 -> [_ w447]
              tunnel: w420 -> [_ w446]
              tunnel: w421 -> [_ w445]
              frame False {
              }
              frame True {
                n154 = for {
                  tunnel: w450 -> [_]
                  tunnel: w449 -> [w457] mode=indexing
                  shift-right: [w458] -> w451
                  shift-left: w448 -> [w456]
                  tunnel: w447 -> [_]
                  tunnel: w446 -> [w455]
                  tunnel: w445 -> [w454]
                  n155 = case shown="0, Default" w457 {
                    tunnel: [w466 w467] -> w453
                    tunnel: w455 -> [_ w467]
                    tunnel: w454 -> [w466 _]
                    frame 0, Default {
                    }
                    frame 1 {
                    }
                  }
                  n156 = Number To Decimal String(number=w457) -> (decimal integer string=w460:string)  [unwired: 1 in]
                  n157 = Concatenate Strings("CamAndor" ("string"), w460) -> (w459:string)
                  n158 = To Long Integer(number=w453) -> (32bit integer=w452:i32[][])
                  n159 = Obtain Queue(name (unnamed)=w459, element data type="Intensity DataInit", create if not found? (T)=FALSE, error in (no error)=w456) -> (queue out=w465:refnum<queue>, error out=w464:errorcluster)  [unwired: 1 in, 1 out]
                  n160 = Lossy Enqueue Element(queue=w465, element=w452, error in (no error)=w464) -> (error out=w458:errorcluster)  [unwired: 3 out]
                }
              }
            }
            "z num" <- w433
            "z vorgabe" <- w441
          }
          n161 = call "ShutDownTimingDIO_ScannerStage.vi"("task out 7"=w227, "error IO"=w233, "task out 2"=w232, "task out 3"=w231, "task out 5"=w229, "task out 9"=w226, "task out"=w224, "task out 10"=w225, "task out 6"=w228, "task out 4"=w230) -> ()  [unwired: 9 in, 1 out]
          n162 = Bundle By Name(cluster="PictureInfo", "Sum_X"=w300, "Sum_Y"=w299, "Pos_X"=w275, "Pos_Y"=w298, "Pos_Z"=w270, "Image_Size_X"=w273, "Image_Size_Y"=w271) -> (w297:T3)
          n163 = call <vilib>:"DAQmx Clear Task.vi"("task in"=w308, "error in"=w310) -> ("error out"=w282:errorcluster)  [unwired: 13 in]
          n164 = call <vilib>:"DAQmx Clear Task.vi"("task in"=w284, "error in"=w282) -> ("error out"=w283:errorcluster)  [unwired: 13 in]
          n165 = call <vilib>:"General Error Handler.vi"("type of dialog (OK msg:1)"=w307, "error in (no error)"=w283) -> ("error out"=w313:errorcluster)  [unwired: 9 in, 4 out]
          n166 = call <vilib>:"DAQmx Clear Task.vi"("task in"=w309, "error in"=w313) -> ("error out"=w311:errorcluster)  [unwired: 13 in]
          n167 = call <vilib>:"General Error Handler.vi"("type of dialog (OK msg:1)"=w312, "error in (no error)"=w311) -> ("error out"=w262:errorcluster)  [unwired: 9 in, 4 out]
          n168 = Bundle(cluster="Binning", "Horizontal bin"=w293, "Vertical bin"=w292) -> (w291:T4)
          n169 = for {
            N: w305 -> [_]
            tunnel: w264 -> [w410] mode=indexing
            shift-right: [w418] -> w304
            shift-left: w262 -> [w419]
            tunnel: w297 -> [w415]
            tunnel: w296 -> [w417]
            tunnel: [w414] -> w303
            tunnel: w210 -> [w413]
            tunnel: [w413] -> w295
            tunnel: w291 -> [w412]
            tunnel: "Intensitätsdiode" -> [w411]
            n170 = Bundle By Name(cluster=w415, "Cam_Num"=1) -> (w414:T3)
            n171 = call "Picture_shr_Save_to_matlab.vi"("DataIn"=w410, "Intensität"=w411, "Binning"=w412, "ROI Coordinates In"=w413, "PictureInfo"=w414, "error in"=w419, "SavingMode"=w417) -> ("error out"=w418:errorcluster)  [unwired: 8 in]
          }
          n172 = for {
            N: w305 -> [_]
            shift-right: [w408] -> w261
            shift-left: w304 -> [w409]
            tunnel: w303 -> [w405]
            tunnel: w296 -> [w407]
            tunnel: w295 -> [w403]
            tunnel: w291 -> [w402]
            tunnel: "Intensitätsdiode" -> [w401]
            tunnel: w263 -> [w400] mode=indexing
            n173 = Bundle By Name(cluster=w405, "Cam_Num"=2) -> (w404:T3)
            n174 = call "Picture_shr_Save_to_matlab.vi"("DataIn"=w400, "Intensität"=w401, "Binning"=w402, "ROI Coordinates In"=w403, "PictureInfo"=w404, "error in"=w409, "SavingMode"=w407) -> ("error out"=w408:errorcluster)  [unwired: 8 in]
          }
        }
      }
    }
  }
  "error out" <- w21
